vi "LoadInstrConfig_LS1.vi"(8 "error in (no error)":errorcluster caption="entrée d'erreur", 10 "Experiment":path, 11 "LoadExp":bool=TRUE) -> (0 "error out":errorcluster caption="sortie d'erreur", 2 "LoadExper Out":bool, 3 "Experiment.lvclass":refnum<class "Experiment.lvclass">)   [LabVIEW 2010]
uses:
  Experiment Class/Experiment.lvclass
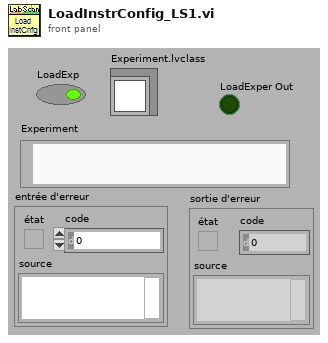
[diagram p1: front panel]
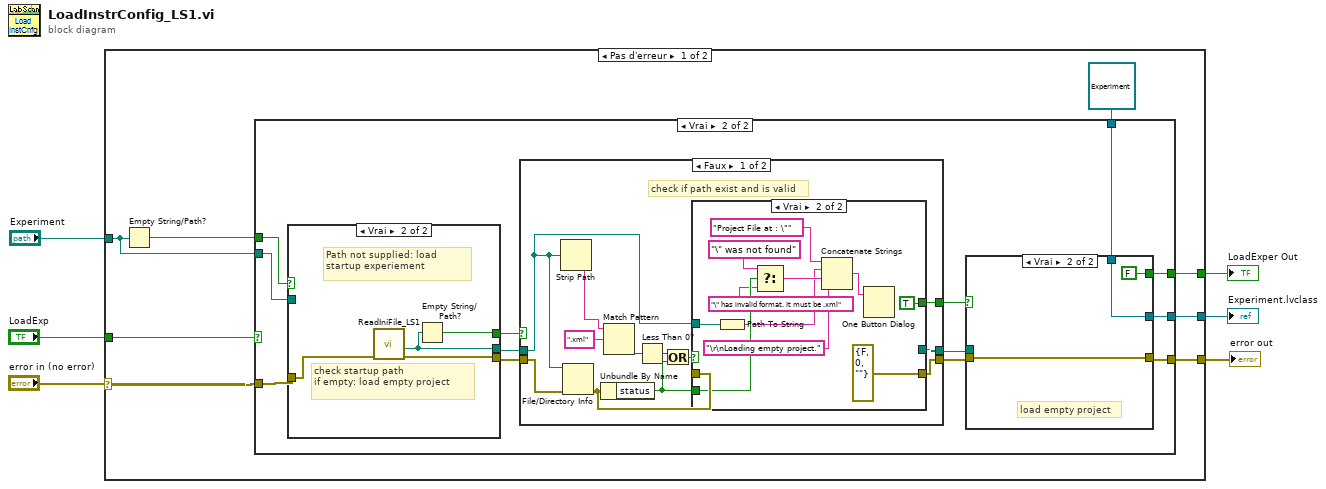
[diagram p0: block diagram]
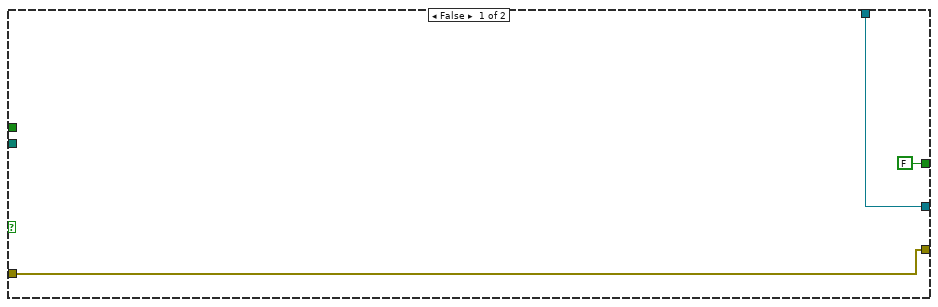
[diagram p2: hidden frame]
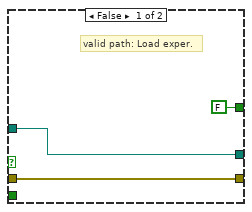
[diagram p3: hidden frame]
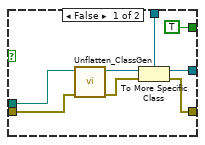
[diagram p6: hidden frame]
diagram:
  n1 = case shown="Pas d'erreur" "error in (no error)" {
    selector: "error in (no error)" -> [w14 w78]
    tunnel: [w11 w78] -> w6
    tunnel: [w13 _] -> w4
    tunnel: "LoadExp" -> [w10 _]
    tunnel: "Experiment" -> [w8 _]
    tunnel: [w7 _] -> w1
    frame No Error {
      n2 = Empty String/Path?(string/path=w8) -> (empty?=w9:bool)
      n3 = case shown="Vrai" w10 {
        tunnel: w14 -> [w16 w27]
        tunnel: [w17 w30] -> w13
        tunnel: refnum<class "Experiment.lvclass"> refnum ("Experiment.lvclass") -> [w17 w29]
        tunnel: [w16 w28] -> w11
        tunnel: w9 -> [_ w26]
        tunnel: w8 -> [_ w20]
        tunnel: [FALSE w18] -> w7
        frame False {
        }
        frame True {
          n4 = case shown="Vrai" w26 {
            selector: w26 -> [w60 _]
            tunnel: w27 -> [w62 w66]
            tunnel: [w62 w65] -> w23
            tunnel: [w60 w64] -> w25
            tunnel: [w61 w63] -> w22
            tunnel: w20 -> [w61 _]
            frame False {
              # "Path supplied\nLoad from that path"
            }
            frame True {
              # "check startup path\nif empty: load empty project"
              # "Path not supplied: load startup experiement"
              n5 = call "ReadIniFile_LS1.vi"("Error in"=w66) -> ("Error out"=w65:errorcluster, "Experiment"=w63:path)  [unwired: 5 in, 4 out]
              n6 = Empty String/Path?(string/path=w63) -> (empty?=w64:bool)
            }
          }
          n7 = case shown="Faux" w25 {
            selector: w25 -> [_ w57]
            tunnel: [w34 w59] -> w24
            tunnel: w23 -> [w40 w59]
            tunnel: w22 -> [w35 w58]
            tunnel: [w36 w58] -> w21
            tunnel: [w31 w57] -> w19
            frame False {
              # "check if path exist and is valid"
              n8 = Strip Path(path=w35) -> (name=w41:string)  [unwired: 1 out]
              n9 = File/Directory Info(path=w35, error in=w40) -> (error out=w33:errorcluster)  [unwired: 6 out]
              n10 = Unbundle By Name(w33) -> ("status"=w32:bool)
              n11 = Match Pattern(string=w41, regular expression=".xml" ("expression régulière")) -> (offset past match=w38:i32)  [unwired: 1 in, 3 out]
              n12 = Less Than 0?(x=w38) -> (x < 0?=w39:bool)
              n13 = Or(x=w39, y=w32) -> (x .or. y?=w37:bool)
              n14 = case shown="Vrai" w37 {
                tunnel: [w45 _] -> w36
                tunnel: w35 -> [w45 w55]
                tunnel: [w44 errorcluster {"status"=FALSE, "code"=0, "source"=""} ("error out")] -> w34
                tunnel: w33 -> [w44 _]
                tunnel: w32 -> [_ w54]
                tunnel: [FALSE ("true") TRUE ("true")] -> w31
                frame False {
                  # "valid path: Load exper."
                }
                frame True {
                  n15 = Path To String(path=w55) -> (string=w49:string)
                  n16 = Select(t="\" was not found" ("message"), s=w54, f="\" has invalid format. It must be .xml" ("message")) -> (s? t:f=w51:string)
                  n17 = Concatenate Strings("Project File at : \"" ("message"), w49, w51, "\r\nLoading empty project." ("message")) -> (w48:string)
                  n18 = One Button Dialog(message=w48) -> ()  [unwired: 1 in, 1 out]
                }
              }
            }
            frame True {
              # "empty startup path"
            }
          }
          n19 = case shown="Vrai" w19 {
            tunnel: [w74 w77] -> w30
            tunnel: w29 -> [w73 w77]
            tunnel: [w72 w76] -> w28
            tunnel: w24 -> [w70 w76]
            tunnel: w21 -> [w69 _]
            tunnel: [TRUE FALSE] -> w18
            frame False {
              n20 = call <userlib>:"Unflatten_ClassGen.vi"("error in (no error)"=w70, "XML File Path"=w69) -> ("sortie d'erreur"=w68:errorcluster, "LabVIEW Object"=w71:refnum<class>)  [unwired: 8 in]
              n21 = To More Specific Class(target class=w73, reference=w71, error in=w68) -> (specific class reference=w74:refnum<class "Experiment.lvclass">, error out=w72:errorcluster)
            }
            frame True {
              # "load empty project"
            }
          }
        }
      }
    }
    frame Error {
    }
  }
  "error out" <- w6
  "Experiment.lvclass" <- w4
  "LoadExper Out" <- w1
